vi "Begin.vi"() -> (1 "CameraDevRef":T5)   [LabVIEW 2011]
doc: "Called before other user functions, this VI is expected to open initial I/O refnums, load in file data, and do all program initialization. Notice that the <B>error out</B> terminal is simply used for data flow. Wiring it to other structures or subVIs ensures that this VI runs first."
uses:
  <vilib>/Rock Robotics/WPI/Camera/WPI_CameraDevRef.ctl
  <vilib>/Rock Robotics/WPI/Encoder/WPI_EncoderDevRef.ctl
  <vilib>/Rock Robotics/SystemInterfaces/Encoder/FPGA_EncoderIdx.ctl
  <vilib>/Rock Robotics/SystemInterfaces/Counter/FPGA_CounterCtrSystemIndex.ctl
  <vilib>/Rock Robotics/WPI/Encoder/WPI_EncoderType.ctl
  <vilib>/Rock Robotics/WPI/Joystick/WPI_JoystickDeviceEnum.ctl
  <vilib>/Rock Robotics/SystemInterfaces/DIO/FPGA_DIOPWMChannel.ctl
  <vilib>/Rock Robotics/SystemInterfaces/Typedef/FPGA_TypedefDigitalModule.ctl
  <vilib>/Rock Robotics/SystemInterfaces/DIO/FPGA_DIOChannel.ctl
  <vilib>/Rock Robotics/SystemInterfaces/AI/FPGA_AIChannel.ctl
  <vilib>/Rock Robotics/WPI/MotorControl/WPI_MotorControlOpen Victor.vi
  <vilib>/Rock Robotics/WPI/Counter/WPI_CounterDigitalInputToDigitalSource.vi
  Robot Global Data.vi
  <vilib>/Rock Robotics/WPI/MotorControl/WPI_MotorControlOpen Jaguar.vi
  <vilib>/Utility/file.llb/Read From Spreadsheet File (DBL).vi
  <vilib>/Rock Robotics/SystemInterfaces/DIO/FPGA_DIORelayChannel.ctl
  <vilib>/Rock Robotics/WPI/Relay/WPI_RelayDirection.ctl
  <vilib>/Rock Robotics/SystemInterfaces/AI/FPGA_AIGyroChannel.ctl
  <vilib>/Rock Robotics/SystemInterfaces/Typedef/FPGA_TypedefAnalogModule.ctl
panel:
  out "Path and file":string
  in  "Balls In Robot At Start":dbl=2.0
  out "EncoderDevRef 2":T1={"DevStatus"={"status"=FALSE, "code"=0, "source"=""}, "EncoderIndex"=enum."Invalid", "CounterIndex"=enum."Invalid", "DistancePerCount"=1.0, "Decoding Type"=enum."4x"}
  out "LDriveEncoder 2":errorcluster
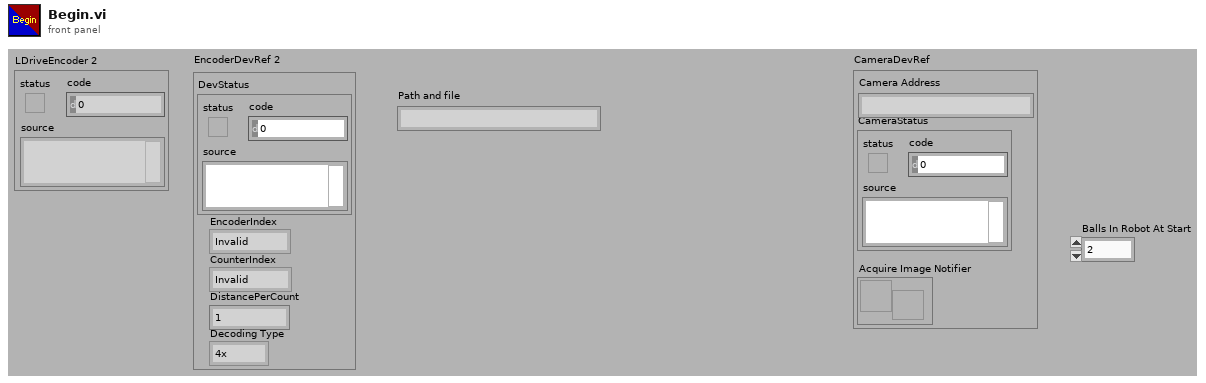
[diagram p1: front panel]
types:
  T1 = typedef "WPI_EncoderDevRef.ctl" = cluster{"DevStatus":errorcluster, "EncoderIndex":T2, "CounterIndex":T3, "DistancePerCount":dbl, "Decoding Type":T4}
  T2 = typedef "FPGA_EncoderIdx.ctl" = enum8{"Enc 0", "Enc 1", "Enc 2", "Enc 3", "Invalid"}
  T3 = typedef "FPGA_CounterCtrSystemIndex.ctl" = enum8{"Ctr 0", "Ctr 1", "Ctr 2", "Ctr 3", "Ctr 4", "Ctr 5", "Ctr 6", "Ctr 7", "Invalid"}
  T4 = typedef "WPI_EncoderType.ctl" = enum16{"1x", "2x", "4x"}
  T5 = typedef "WPI_CameraDevRef.ctl" = cluster{"Camera Address":string, "CameraStatus":errorcluster, "Acquire Image Notifier":refnum<notifier>}
  T6 = typedef "FPGA_DIOChannel.ctl" = enum8{"DIO 1", "DIO 2", "DIO 3", "DIO 4", "DIO 5", "DIO 6", "DIO 7", "DIO 8", "DIO 9", "DIO 10", "DIO 11", "DIO 12", "DIO 13", "DIO 14", "Invalid"}
  T7 = typedef "FPGA_DIOPWMChannel.ctl" = enum8{"PWM 1", "PWM 2", "PWM 3", "PWM 4", "PWM 5", "PWM 6", "PWM 7", "PWM 8", "PWM 9", "PWM 10", "Invalid"}
  T8 = typedef "FPGA_AIChannel.ctl" = enum8{"AI 1", "AI 2", "AI 3", "AI 4", "AI 5", "AI 6", "AI 7", "AI 8", "Invalid"}
  T9 = typedef "WPI_JoystickDeviceEnum.ctl" = enum16{"USB 1", "USB 2", "USB 3", "USB 4", "Kinect 1", "Kinect 2"}
  T10 = typedef "FPGA_TypedefDigitalModule.ctl" = enum16{"Digital Module 1", "Digital Module 2"}
  T11 = typedef "WPI_MotorControlDeviceRef.ctl" = cluster{"DeviceStatus":errorcluster, "Type":enum16{"PWM", "CAN"}, "PWM":cluster{"Digital Module":T10, "PWM Channel":T7, "DeadBand":T12}, "CAN":cluster{"Device Number":u8, "Control Mode":T13, "Semaphore":T14, "Max Vout":dbl}, "Invert":bool, "TransformRef":T15, "InvTransformRef":T15}
  T12 = typedef "WPI_PWMDeadband.ctl" = cluster{"Name":string, "maxPositivePwm":i32, "minPositivePwm":i32, "centerPwm":i32, "maxNegativePwm":i32, "minNegativePwm":i32, "angularRange":u16}
  T13 = typedef "WPI_CANJaguar_ControlMode.ctl" = enum8{"Percent VBus", "Current", "Speed", "Position", "Voltage"}
  T14 = typedef "Semaphore RefNum" = refnum<k1>
  T15 = typedef "WPI_PWMTransform_ConPane.ctl" = refnum<vi>
  T16 = typedef "WPI_CameraImageSize.ctl" = enum16{"640x480", "320x240", "160x120"}
  T17 = cluster{"fps":i32, "compression":i32, "Image Size":T16}
  T18 = typedef "WPI_CameraWhite Balance Values.ctl" = enum16{"Auto", "Fixed indoor", "Fixed outdoor 1", "Fixed outdoor 2", "Fixed fluorescent 1", "Fixed fluorescent 2", "Hold current"}
  T19 = typedef "WPI_CameraExposure Values.ctl" = enum16{"Auto", "Flicker-free 50 Hz", "Flicker-free 60 Hz", "Hold current"}
  T20 = typedef "WPI_ServoDeviceRef.ctl" = cluster{"DeviceStatus":errorcluster, "Digital Module":T10, "PWM Channel":T7, "DeadBand":T12}
  T21 = typedef "WPI_DigitalInputDevRef.ctl" = cluster{"DevStatus":errorcluster, "DIO Channel":T6, "Digital Module":T10}
  T22 = typedef "WPI_JoystickDevRef.ctl" = cluster{"Device":T9}
  T23 = typedef "FPGA_CounterEncoderSourceConvertionLVSourceType.ctl" = cluster{"DevStatus":errorcluster, "AnalogTriggerMode?":bool, "DigitalMode":cluster{"Digital Module":T10, "DIO Channel":T24}, "AnalogTriggerMode":cluster{"AnalogTriggerIndex":T25, "OutputType":T26}}
  T24 = typedef "FPGA_DIODigitalSourceChannel.ctl" = enum8{"DIO 1", "DIO 2", "DIO 3", "DIO 4", "DIO 5", "DIO 6", "DIO 7", "DIO 8", "DIO 9", "DIO 10", "DIO 11", "DIO 12", "DIO 13", "DIO 14", "Disabled"}
  T25 = typedef "FPGA_AnalogTriggerIndex.ctl" = enum8{"Trig 0", "Trig 1", "Trig 2", "Trig 3", "Trig 4", "Trig 5", "Trig 6", "Trig 7", "Invalid"}
  T26 = typedef "FPGA_AnalogTriggerOutType.ctl" = enum16{"InWindow", "TriggerState", "Rising", "Falling"}
  T27 = typedef "FPGA_DIORelayChannel.ctl" = enum8{"Relay 1", "Relay 2", "Relay 3", "Relay 4", "Relay 5", "Relay 6", "Relay 7", "Relay 8", "Invalid"}
  T28 = typedef "WPI_RelayDirection.ctl" = enum16{"Both directions", "Forward only", "Reverse only"}
  T29 = typedef "WPI_AnalogChannelDevRef.ctl" = cluster{"DevStatus":errorcluster, "Analog Module":T30, "Analog Channel":T8}
  T30 = typedef "FPGA_TypedefAnalogModule.ctl" = enum16{"Analog Module 1", "Analog Module 2"}
  T31 = typedef "WPI_RelayDevRef.ctl" = cluster{"DevStatus":errorcluster, "Relay Channel":T27, "Digital Module":T10, "Relay Direction":T28}
  T32 = typedef "FPGA_AIGyroChannel.ctl" = enum8{"AI 1", "AI 2", "Invalid"}
  T33 = typedef "WPI_GyroDevRef.ctl" = cluster{"DevStatus":errorcluster, "Analog Module":T30, "Analog Channel":T8, "Offset":dbl, "Gain (VoltsPerDegree/Second)":dbl}
  T34 = typedef "WPI_UltrasonicDeviceRef.ctl" = cluster{"DevStatus":errorcluster, "Ping Digital Module":T10, "Echo Digital Module":T10, "Ping Channel":T6, "Echo Channel":T6, "CntIndex":T3}
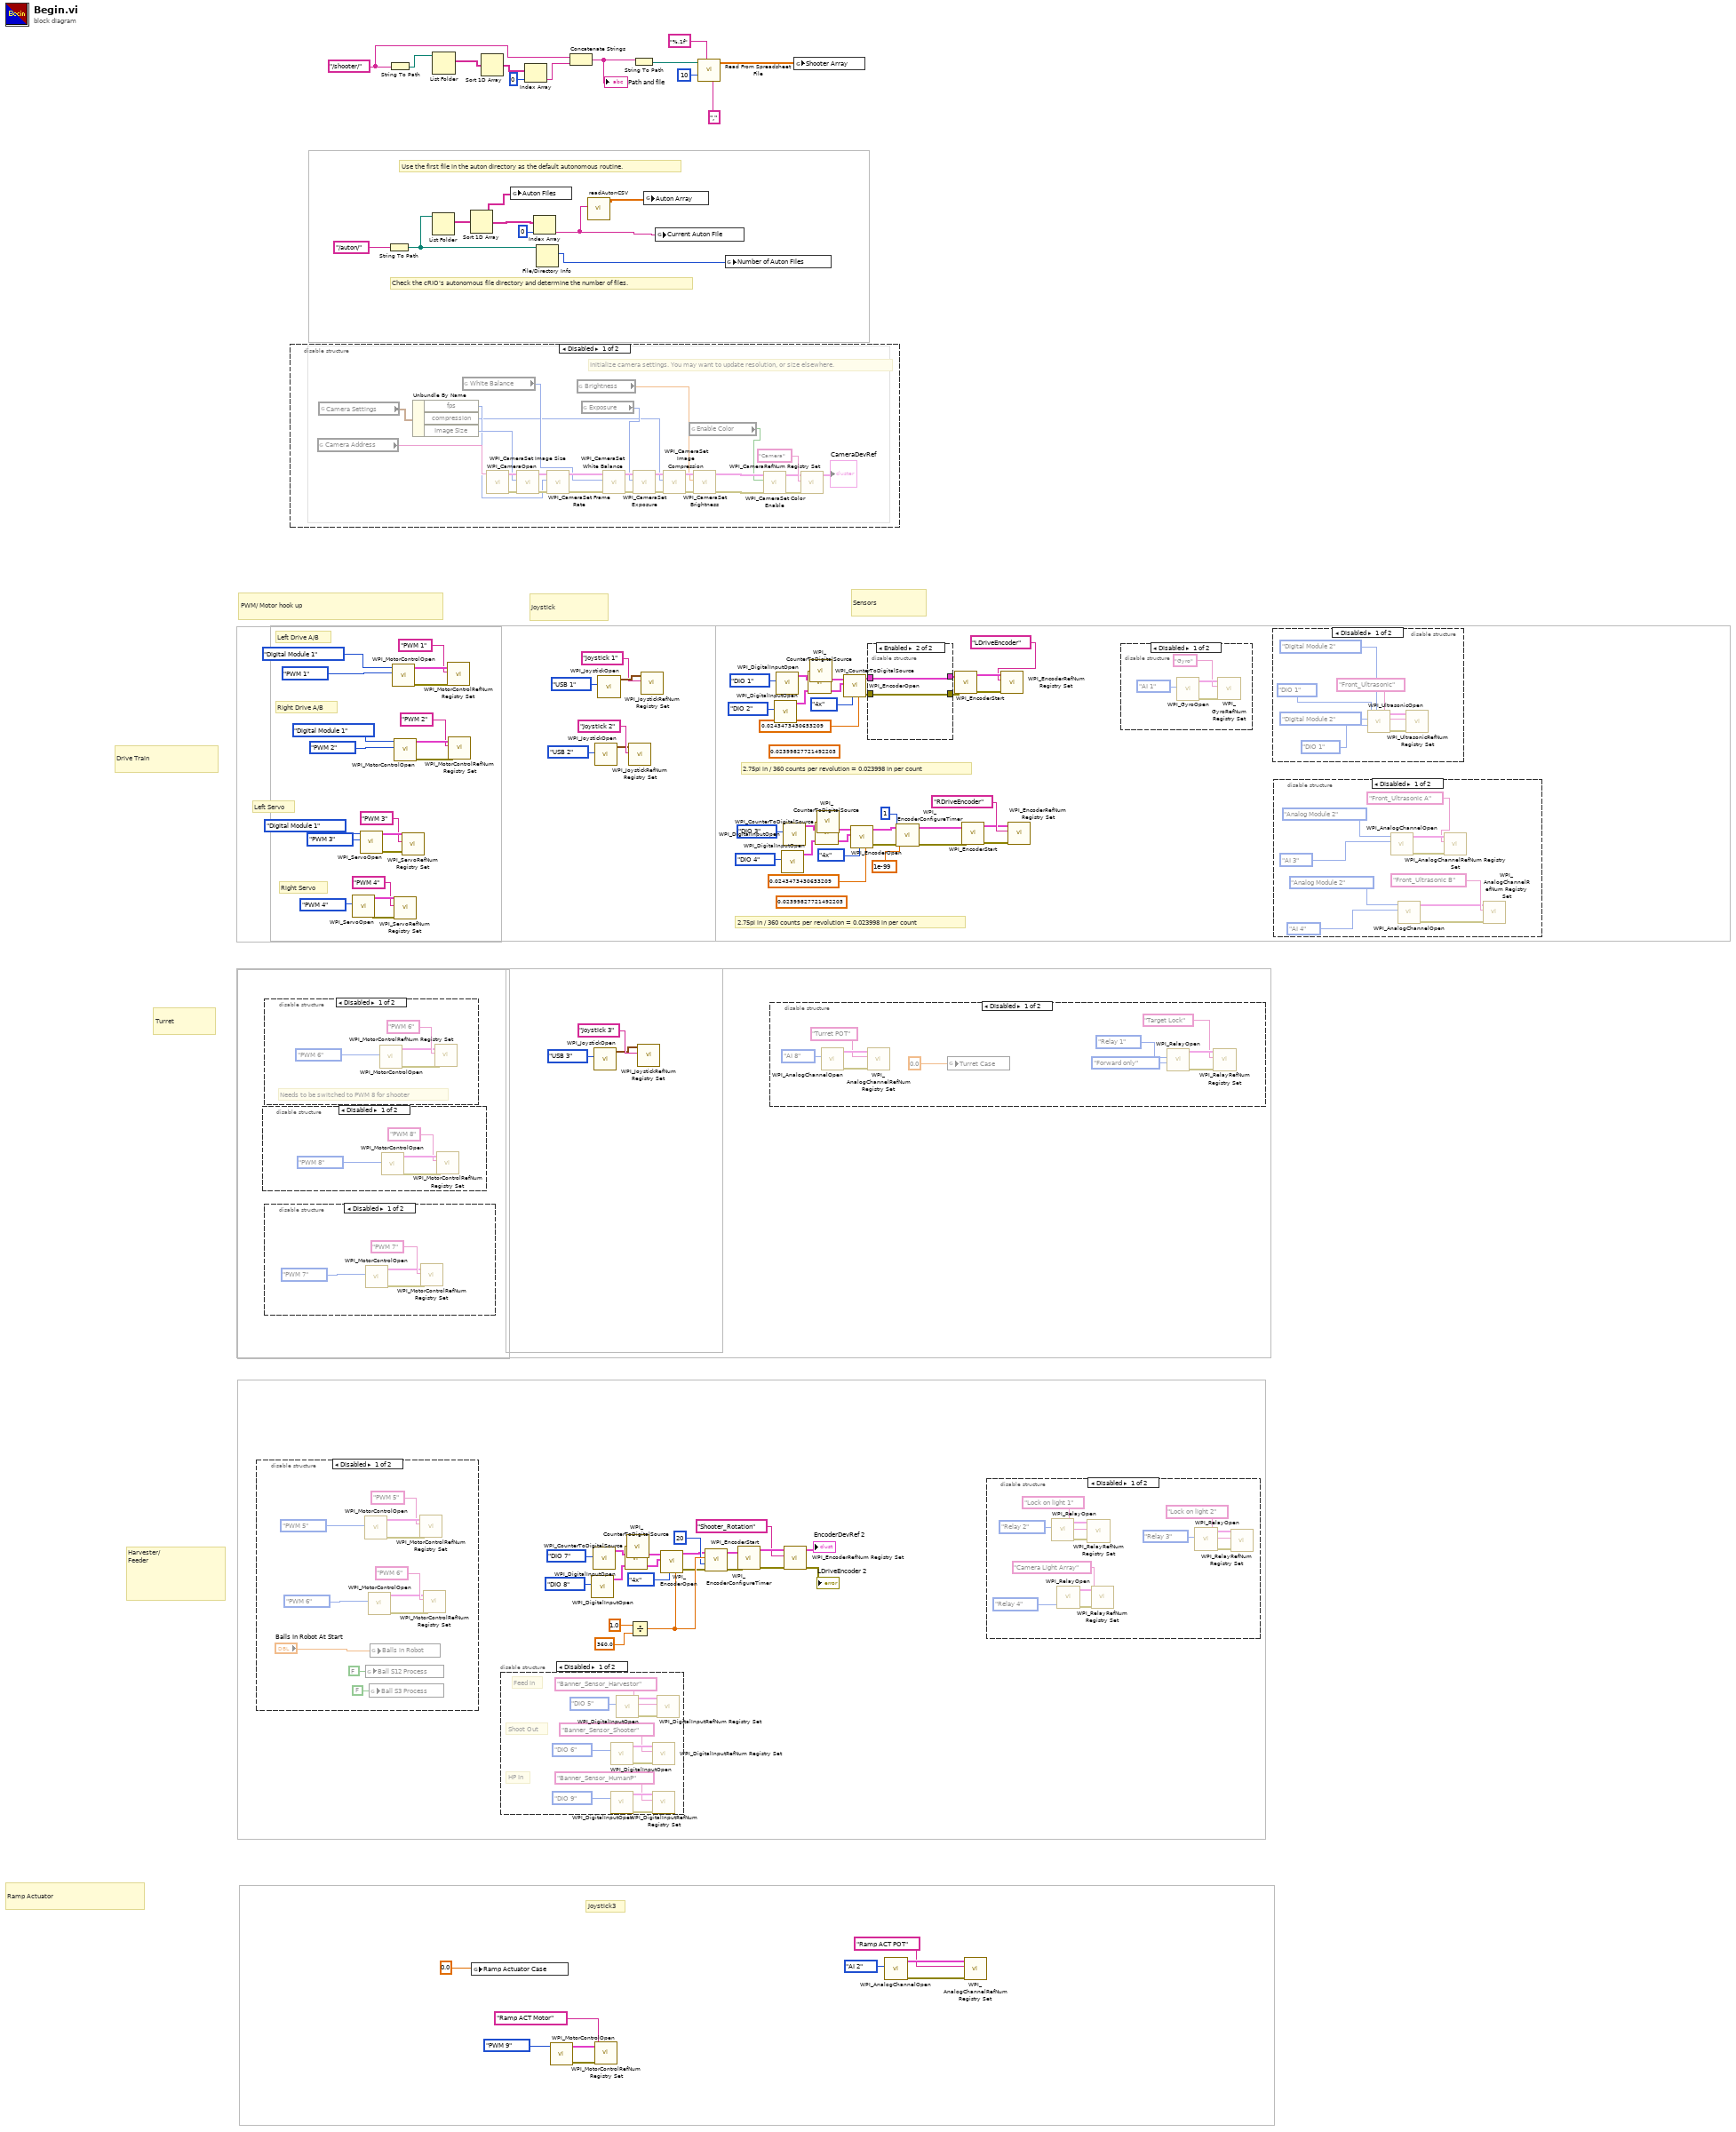
[diagram p0: block diagram]
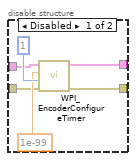
[diagram p2: hidden frame]
diagram:
  w26 = "/shooter/" ("string")
  (unwired) 0.02399827721492203 ("DistancePerCount")
  (unwired) 0.02399827721492203 ("DistancePerCount")
  # "2.75pi in / 360 counts per revolution = 0.023998 in per count"
  # "2.75pi in / 360 counts per revolution = 0.023998 in per count"
  # "Joystick3"
  # "Check the cRIO's autonomous file directory and determine the number of files."
  # "Use the first file in the auton directory as the default autonomous routine."
  # "Harvester/\nFeeder"
  # "Right Drive A/B"
  # "Left Drive A/B"
  # "Right Servo"
  # "Left Servo"
  # "Turret"
  # "Ramp Actuator"
  # "Drive Train"
  # "Sensors"
  # "Joystick"
  # "PWM/ Motor hook up"
  n1 = disable-structure shown="Disabled" {
    frame Disabled {
      n2 = call-poly <vilib>:"WPI_MotorControlOpen.vi"("PWM Channel"=FPGA_DIOPWMChannel."PWM 5") -> ("error out"=w117:errorcluster, "MotorControlDeviceRef"=w119:T11)  [unwired: 9 in]
      n3 = global write "Robot Global Data.vi" "Ball S12 Process"(FALSE ("Ball S12 Process")) -> ()
      n4 = call-poly <vilib>:"WPI_MotorControlOpen.vi"("PWM Channel"=FPGA_DIOPWMChannel."PWM 6") -> ("error out"=w116:errorcluster, "MotorControlDeviceRef"=w114:T11)  [unwired: 9 in]
      n5 = global write "Robot Global Data.vi" "Ball S3 Process"(FALSE ("Ball S3 Process")) -> ()
      n6 = global write "Robot Global Data.vi" "Balls in Robot"("Balls In Robot At Start") -> ()
      n7 = call <vilib>:"WPI_MotorControlRefNum Registry Set.vi"("error in (no error)"=w117, "refnum name"="PWM 5", "MotorControlDevRef"=w119) -> ()  [unwired: 7 in, 2 out]
      n8 = call <vilib>:"WPI_MotorControlRefNum Registry Set.vi"("error in (no error)"=w116, "refnum name"="PWM 6", "MotorControlDevRef"=w114) -> ()  [unwired: 7 in, 2 out]
    }
    frame Enabled {
    }
  }
  n9 = disable-structure shown="Disabled" {
    frame Disabled {
      n10 = call-poly <vilib>:"WPI_MotorControlOpen.vi"("PWM Channel"=FPGA_DIOPWMChannel."PWM 8") -> ("error out"=w121:errorcluster, "MotorControlDeviceRef"=w123:T11)  [unwired: 9 in]
      n11 = call <vilib>:"WPI_MotorControlRefNum Registry Set.vi"("error in (no error)"=w121, "refnum name"="PWM 8", "MotorControlDevRef"=w123) -> ()  [unwired: 7 in, 2 out]
    }
    frame Enabled {
    }
  }
  n12 = disable-structure shown="Disabled" {
    frame Disabled {
      # "Needs to be switched to PWM 8 for shooter"
      n13 = call-poly <vilib>:"WPI_MotorControlOpen.vi"("PWM Channel"=FPGA_DIOPWMChannel."PWM 6") -> ("error out"=w128:errorcluster, "MotorControlDeviceRef"=w126:T11)  [unwired: 9 in]
      n14 = call <vilib>:"WPI_MotorControlRefNum Registry Set.vi"("error in (no error)"=w128, "refnum name"="PWM 6", "MotorControlDevRef"=w126) -> ()  [unwired: 7 in, 2 out]
    }
    frame Enabled {
    }
  }
  n15 = disable-structure shown="Disabled" {
    frame Disabled {
      n16 = call-poly <vilib>:"WPI_MotorControlOpen.vi"("PWM Channel"=FPGA_DIOPWMChannel."PWM 7") -> ("error out"=w132:errorcluster, "MotorControlDeviceRef"=w130:T11)  [unwired: 9 in]
      n17 = call <vilib>:"WPI_MotorControlRefNum Registry Set.vi"("error in (no error)"=w132, "refnum name"="PWM 7", "MotorControlDevRef"=w130) -> ()  [unwired: 7 in, 2 out]
    }
    frame Enabled {
    }
  }
  n18 = disable-structure shown="Disabled" {
    frame Disabled {
      # "Initialize camera settings. You may want to update resolution, or size elsewhere."
      n19 = global read "Robot Global Data.vi" "Camera Address"() -> (w146:string)
      n20 = global read "Robot Global Data.vi" "Camera Settings"() -> (w145:T17)
      n21 = Unbundle By Name(w145) -> ("fps"=w143:i32, "compression"=w140:i32, "Image Size"=w144:T16)
      n22 = global read "Robot Global Data.vi" "White Balance"() -> (w142:T18)
      n23 = call <vilib>:"WPI_CameraOpen.vi"("Camera Address"=w146) -> ("error out"=w152:errorcluster, "CameraDevRef"=w153:T5)  [unwired: 1 in, 8 out]
      n24 = call <vilib>:"WPI_CameraSet Image Size.vi"("error in (no error)"=w152, "Image Size"=w144, "CameraDevRef"=w153) -> ("error out"=w151:errorcluster, "CameraDevRef Out"=w154:T5)  [unwired: 7 out]
      n25 = call <vilib>:"WPI_CameraSet Frame Rate.vi"("error in (no error)"=w151, "Frame Rate (fps)"=w143, "CameraDevRef"=w154) -> ("error out"=w150:errorcluster, "CameraDevRef Out"=w156:T5)  [unwired: 7 out]
      n26 = global read "Robot Global Data.vi" "Brightness"() -> (w139:dbl)
      n27 = global read "Robot Global Data.vi" "Exposure"() -> (w141:T19)
      n28 = call <vilib>:"WPI_CameraSet White Balance.vi"("error in (no error)"=w150, "White Balance"=w142, "CameraDevRef"=w156) -> ("error out"=w149:errorcluster, "CameraDevRef Out"=w155:T5)  [unwired: 7 out]
      n29 = call <vilib>:"WPI_CameraSet Exposure.vi"("error in (no error)"=w149, "Exposure"=w141, "CameraDevRef"=w155) -> ("error out"=w148:errorcluster, "CameraDevRef Out"=w158:T5)  [unwired: 7 out]
      n30 = call <vilib>:"WPI_CameraSet Image Compression.vi"("error in (no error)"=w148, "Compression"=w140, "CameraDevRef"=w158) -> ("error out"=w147:errorcluster, "CameraDevRef Out"=w157:T5)  [unwired: 7 out]
      n31 = global read "Robot Global Data.vi" "Enable Color"() -> (w134:bool)
      n32 = call <vilib>:"WPI_CameraSet Brightness.vi"("error in (no error)"=w147, "Brightness"=w139, "CameraDevRef"=w157) -> ("error out"=w137:errorcluster, "CameraDevRef Out"=w138:T5)  [unwired: 7 out]
      n33 = call <vilib>:"WPI_CameraSet Color Enable.vi"("error in (no error)"=w137, "Color Enabled"=w134, "CameraDevRef"=w138) -> ("error out"=w135:errorcluster, "CameraDevRef Out"=w136:T5)  [unwired: 7 in]
      n34 = call <vilib>:"WPI_CameraRefNum Registry Set.vi"("error in (no error)"=w135, "refnum name"="Camera", "CameraDevRef"=w136) -> ("CameraDevRef"=→"CameraDevRef":T5)  [unwired: 8 out]
    }
    frame Enabled {
    }
  }
  n35 = call <vilib>:"WPI_ServoOpen.vi"("PWM Channel"=FPGA_DIOPWMChannel."PWM 4") -> ("error out"=w85:errorcluster, "ServoDeviceRef"=w100:T20)  [unwired: 9 in]
  n36 = call <vilib>:"WPI_ServoOpen.vi"("PWM Channel"=FPGA_DIOPWMChannel."PWM 3", "Digital Module (Module 1)"=FPGA_TypedefDigitalModule."Digital Module 1") -> ("error out"=w86:errorcluster, "ServoDeviceRef"=w102:T20)  [unwired: 8 in]
  n37 = String To Path(string="/auton/") -> (path=w54:path)
  n38 = String To Path(string=w26) -> (path=w35:path)
  n39 = call-poly <vilib>:"WPI_MotorControlOpen.vi"("PWM Channel"=FPGA_DIOPWMChannel."PWM 1", "Digital Module (Module 1)"=FPGA_TypedefDigitalModule."Digital Module 1") -> ("error out"=w90:errorcluster, "MotorControlDeviceRef"=w93:T11)  [unwired: 8 in]
  n40 = call-poly <vilib>:"WPI_MotorControlOpen.vi"("PWM Channel"=FPGA_DIOPWMChannel."PWM 2", "Digital Module (Module 1)"=FPGA_TypedefDigitalModule."Digital Module 1") -> ("error out"=w91:errorcluster, "MotorControlDeviceRef"=w96:T11)  [unwired: 8 in]
  n41 = call <vilib>:"WPI_ServoRefNum Registry Set.vi"("error in (no error)"=w85, "refnum name"="PWM 4", "ServoDeviceRef"=w100) -> ()  [unwired: 7 in, 2 out]
  n42 = call <vilib>:"WPI_ServoRefNum Registry Set.vi"("error in (no error)"=w86, "refnum name"="PWM 3", "ServoDeviceRef"=w102) -> ()  [unwired: 7 in, 2 out]
  n43 = List Folder(path=w54) -> (filenames=w53:string[])  [unwired: 1 in, 5 out]
  n44 = List Folder(path=w35) -> (filenames=w34:string[])  [unwired: 1 in, 5 out]
  n45 = call <vilib>:"WPI_MotorControlRefNum Registry Set.vi"("error in (no error)"=w90, "refnum name"="PWM 1", "MotorControlDevRef"=w93) -> ()  [unwired: 7 in, 2 out]
  n46 = call <vilib>:"WPI_MotorControlRefNum Registry Set.vi"("error in (no error)"=w91, "refnum name"="PWM 2", "MotorControlDevRef"=w96) -> ()  [unwired: 7 in, 2 out]
  n47 = Sort 1D Array(array=w53) -> (sorted array=w48:string[])
  n48 = global write "Robot Global Data.vi" "Ramp Actuator Case"(0.0 ("Ramp Actuator Case")) -> ()
  n49 = Sort 1D Array(array=w34) -> (sorted array=w33:string[])
  n50 = disable-structure shown="Disabled" {
    frame Disabled {
      # "HP In"
      # "Shoot Out"
      # "Feed in"
      n51 = call <vilib>:"WPI_DigitalInputOpen.vi"("DIO Channel"=FPGA_DIOChannel."DIO 6") -> ("error out"=w166:errorcluster, "DigitalInputDevRef"=w165:T21)  [unwired: 9 in]
      n52 = call <vilib>:"WPI_DigitalInputOpen.vi"("DIO Channel"=FPGA_DIOChannel."DIO 9") -> ("error out"=w162:errorcluster, "DigitalInputDevRef"=w161:T21)  [unwired: 9 in]
      n53 = call <vilib>:"WPI_DigitalInputOpen.vi"("DIO Channel"=FPGA_DIOChannel."DIO 5") -> ("error out"=w169:errorcluster, "DigitalInputDevRef"=w168:T21)  [unwired: 9 in]
      n54 = call <vilib>:"WPI_DigitalInputRefNum Registry Set.vi"("error in (no error)"=w166, "refnum name"="Banner_Sensor_Shooter", "DigitalInputDevRef"=w165) -> ()  [unwired: 7 in, 2 out]
      n55 = call <vilib>:"WPI_DigitalInputRefNum Registry Set.vi"("error in (no error)"=w162, "refnum name"="Banner_Sensor_HumanP", "DigitalInputDevRef"=w161) -> ()  [unwired: 7 in, 2 out]
      n56 = call <vilib>:"WPI_DigitalInputRefNum Registry Set.vi"("error in (no error)"=w169, "refnum name"="Banner_Sensor_Harvestor", "DigitalInputDevRef"=w168) -> ()  [unwired: 7 in, 2 out]
    }
    frame Enabled {
    }
  }
  n57 = global write "Robot Global Data.vi" "Auton Files"(w48) -> ()
  n58 = Index Array(array=w33, index=0) -> (element=w25:string)
  n59 = Index Array(array=w48, index=0) -> (element=w50:string)
  n60 = File/Directory Info(path=w54) -> (size=w51:i64)  [unwired: 1 in, 6 out]
  n61 = call-poly <vilib>:"WPI_MotorControlOpen.vi"("PWM Channel"=FPGA_DIOPWMChannel."PWM 9") -> ("error out"=w38:errorcluster, "MotorControlDeviceRef"=w39:T11)  [unwired: 9 in]
  n62 = Concatenate Strings(w26, w25) -> (w28:string)
  "Path and file" <- w28
  n63 = call "readAutonCSV.vi"("AutonFile"=w50) -> ("AutonArray"=w49:dbl[][])  [unwired: 7 in]
  n64 = call <vilib>:"WPI_DigitalInputOpen.vi"("DIO Channel"=FPGA_DIOChannel."DIO 8") -> ("DigitalInputDevRef"=w8:T21)  [unwired: 9 in, 1 out]
  n65 = call <vilib>:"WPI_DigitalInputOpen.vi"("DIO Channel"=FPGA_DIOChannel."DIO 7") -> ("DigitalInputDevRef"=w5:T21)  [unwired: 9 in, 1 out]
  n66 = call <vilib>:"WPI_JoystickOpen.vi"("JoystickDevice"=WPI_JoystickDeviceEnum."USB 3") -> ("JoystickDevRef"=w46:T22)  [unwired: 10 in]
  n67 = call <vilib>:"WPI_JoystickOpen.vi"("JoystickDevice"=WPI_JoystickDeviceEnum."USB 2") -> ("JoystickDevRef"=w106:T22)  [unwired: 10 in]
  n68 = call <vilib>:"WPI_MotorControlRefNum Registry Set.vi"("error in (no error)"=w38, "refnum name"="Ramp ACT Motor", "MotorControlDevRef"=w39) -> ()  [unwired: 7 in, 2 out]
  n69 = call <vilib>:"WPI_JoystickOpen.vi"("JoystickDevice"=WPI_JoystickDeviceEnum."USB 1") -> ("JoystickDevRef"=w109:T22)  [unwired: 10 in]
  n70 = call-poly <vilib>:"WPI_CounterToDigitalSource.vi"("DigitalInputDevRef"=w8) -> ("Digital Source"=w9:T23)  [unwired: 6 in]
  n71 = call-poly <vilib>:"WPI_CounterToDigitalSource.vi"("DigitalInputDevRef"=w5) -> ("Digital Source"=w4:T23)  [unwired: 6 in]
  n72 = call <vilib>:"WPI_JoystickRefNum Registry Set.vi"("refnum name"="Joystick 2", "JoystickDevRef"=w106) -> ()  [unwired: 8 in, 2 out]
  n73 = Divide(x=1.0, y=360.0) -> (x/y=w23:dbl)
  n74 = String To Path(string=w28) -> (path=w27:path)
  n75 = call <vilib>:"WPI_JoystickRefNum Registry Set.vi"("refnum name"="Joystick 3", "JoystickDevRef"=w46) -> ()  [unwired: 8 in, 2 out]
  n76 = call <vilib>:"WPI_JoystickRefNum Registry Set.vi"("refnum name"="Joystick 1", "JoystickDevRef"=w109) -> ()  [unwired: 8 in, 2 out]
  n77 = global write "Robot Global Data.vi" "Auton Array"(w49) -> ()
  n78 = global write "Robot Global Data.vi" "Current Auton File"(w50) -> ()
  n79 = call <vilib>:"WPI_EncoderOpen.vi"("DistancePerCount"=w23, "Decoding Type"=WPI_EncoderType."4x", "BSource"=w9, "ASource"=w4) -> ("error out"=w12:errorcluster, "EncoderDevRef"=w13:T1)  [unwired: 6 in]
  n80 = call-poly <vilib>:"Read From Spreadsheet File.vi"("delimiter (\\t)"="," ("delimiter (\\t)"), "format (%.3f)"="%.1f", "number of rows (all:-1)"=10, "file path (dialog if empty)"=w27) -> ("all rows"=w24:dbl[][])  [unwired: 1 in, 6 out]
  n81 = call <vilib>:"WPI_EncoderConfigureTimer.vi"("error in (no error)"=w12, "Number Samples to Average"=u8 20, "Minimum Rate"=w23, "EncoderDevRef"=w13) -> ("error out"=w16:errorcluster, "EncoderDevRef"=w15:T1)  [unwired: 6 in]
  n82 = global write "Robot Global Data.vi" "Number of Auton Files"(w51) -> ()
  n83 = call <vilib>:"WPI_EncoderStart.vi"("error in (no error)"=w16, "EncoderDevRef"=w15) -> ("error out"=w18:errorcluster, "EncoderDevRef"=w17:T1)  [unwired: 8 in]
  n84 = disable-structure shown="Disabled" {
    frame Disabled {
      n85 = call <vilib>:"WPI_AnalogChannelOpen.vi"("Analog Channel"=FPGA_AIChannel."AI 8") -> ("error out"=w175:errorcluster, "AIDeviceRef"=w176:T29)  [unwired: 9 in]
      n86 = call <vilib>:"WPI_AnalogChannelRefNum Registry Set.vi"("error in (no error)"=w175, "refnum name"="Turret POT", "AIDeviceRef"=w176) -> ()  [unwired: 7 in, 2 out]
      n87 = global write "Robot Global Data.vi" "Turret Case"(0.0 ("Return To Home Case")) -> ()
      n88 = call <vilib>:"WPI_RelayOpen.vi"("Relay Direction"=WPI_RelayDirection."Forward only", "Relay Channel"=FPGA_DIORelayChannel."Relay 1") -> ("error out"=w180:errorcluster, "RelayDevRef"=w181:T31)  [unwired: 8 in]
      n89 = call <vilib>:"WPI_RelayRefNum Registry Set.vi"("error in (no error)"=w180, "refnum name"="Target Lock", "RelayDevRef"=w181) -> ()  [unwired: 7 in, 2 out]
    }
    frame Enabled {
    }
  }
  n90 = call <vilib>:"WPI_DigitalInputOpen.vi"("DIO Channel"=FPGA_DIOChannel."DIO 2") -> ("DigitalInputDevRef"=w76:T21)  [unwired: 9 in, 1 out]
  n91 = call <vilib>:"WPI_DigitalInputOpen.vi"("DIO Channel"=FPGA_DIOChannel."DIO 1") -> ("DigitalInputDevRef"=w73:T21)  [unwired: 9 in, 1 out]
  n92 = call <vilib>:"WPI_DigitalInputOpen.vi"("DIO Channel"=FPGA_DIOChannel."DIO 4") -> ("DigitalInputDevRef"=w67:T21)  [unwired: 9 in, 1 out]
  n93 = call <vilib>:"WPI_DigitalInputOpen.vi"("DIO Channel"=FPGA_DIOChannel."DIO 3") -> ("DigitalInputDevRef"=w70:T21)  [unwired: 9 in, 1 out]
  n94 = call <vilib>:"WPI_EncoderRefNum Registry Set.vi"("error in (no error)"=w18, "refnum name"="Shooter_Rotation", "EncoderDevRef"=w17) -> ("error out"=→"LDriveEncoder 2":errorcluster, "EncoderDevRef"=→"EncoderDevRef 2":T1)  [unwired: 7 in]
  n95 = global write "Robot Global Data.vi" "Shooter Array"(w24) -> ()
  n96 = call-poly <vilib>:"WPI_CounterToDigitalSource.vi"("DigitalInputDevRef"=w76) -> ("Digital Source"=w77:T23)  [unwired: 6 in]
  n97 = call-poly <vilib>:"WPI_CounterToDigitalSource.vi"("DigitalInputDevRef"=w73) -> ("Digital Source"=w72:T23)  [unwired: 6 in]
  n98 = call-poly <vilib>:"WPI_CounterToDigitalSource.vi"("DigitalInputDevRef"=w67) -> ("Digital Source"=w66:T23)  [unwired: 6 in]
  n99 = call-poly <vilib>:"WPI_CounterToDigitalSource.vi"("DigitalInputDevRef"=w70) -> ("Digital Source"=w71:T23)  [unwired: 6 in]
  n100 = call <vilib>:"WPI_EncoderOpen.vi"("DistancePerCount"=0.0243473430653209, "Decoding Type"=WPI_EncoderType."4x", "BSource"=w77, "ASource"=w72) -> ("error out"=w79:errorcluster, "EncoderDevRef"=w80:T1)  [unwired: 6 in]
  n101 = call <vilib>:"WPI_EncoderOpen.vi"("DistancePerCount"=0.0243473430653209, "Decoding Type"=WPI_EncoderType."4x", "BSource"=w66, "ASource"=w71) -> ("error out"=w63:errorcluster, "EncoderDevRef"=w62:T1)  [unwired: 6 in]
  n102 = disable-structure shown="Enabled" {
    disable-tunnel: [w187 w188] -> w82
    disable-tunnel: [w186 w189] -> w81
    disable-tunnel: w80 -> [w183 w189]
    disable-tunnel: w79 -> [w182 w188]
    frame Disabled {
      n103 = call <vilib>:"WPI_EncoderConfigureTimer.vi"("error in (no error)"=w182, "Number Samples to Average"=u8 1, "Minimum Rate"=1e-99, "EncoderDevRef"=w183) -> ("error out"=w187:errorcluster, "EncoderDevRef"=w186:T1)  [unwired: 6 in]
    }
    frame Enabled {
    }
  }
  n104 = call <vilib>:"WPI_AnalogChannelOpen.vi"("Analog Channel"=FPGA_AIChannel."AI 2") -> ("error out"=w43:errorcluster, "AIDeviceRef"=w44:T29)  [unwired: 9 in]
  n105 = call <vilib>:"WPI_EncoderConfigureTimer.vi"("error in (no error)"=w63, "Number Samples to Average"=u8 1, "Minimum Rate"=1e-99, "EncoderDevRef"=w62) -> ("error out"=w58:errorcluster, "EncoderDevRef"=w59:T1)  [unwired: 6 in]
  n106 = call <vilib>:"WPI_EncoderStart.vi"("error in (no error)"=w82, "EncoderDevRef"=w81) -> ("error out"=w84:errorcluster, "EncoderDevRef"=w83:T1)  [unwired: 8 in]
  n107 = call <vilib>:"WPI_EncoderStart.vi"("error in (no error)"=w58, "EncoderDevRef"=w59) -> ("error out"=w56:errorcluster, "EncoderDevRef"=w57:T1)  [unwired: 8 in]
  n108 = call <vilib>:"WPI_AnalogChannelRefNum Registry Set.vi"("error in (no error)"=w43, "refnum name"="Ramp ACT POT", "AIDeviceRef"=w44) -> ()  [unwired: 7 in, 2 out]
  n109 = disable-structure shown="Disabled" {
    frame Disabled {
      n110 = call <vilib>:"WPI_RelayOpen.vi"("Relay Channel"=FPGA_DIORelayChannel."Relay 2") -> ("error out"=w199:errorcluster, "RelayDevRef"=w198:T31)  [unwired: 9 in]
      n111 = call <vilib>:"WPI_RelayOpen.vi"("Relay Channel"=FPGA_DIORelayChannel."Relay 4") -> ("error out"=w201:errorcluster, "RelayDevRef"=w200:T31)  [unwired: 9 in]
      n112 = call <vilib>:"WPI_RelayRefNum Registry Set.vi"("error in (no error)"=w199, "refnum name"="Lock on light 1", "RelayDevRef"=w198) -> ()  [unwired: 7 in, 2 out]
      n113 = call <vilib>:"WPI_RelayRefNum Registry Set.vi"("error in (no error)"=w201, "refnum name"="Camera Light Array", "RelayDevRef"=w200) -> ()  [unwired: 7 in, 2 out]
      n114 = call <vilib>:"WPI_RelayOpen.vi"("Relay Channel"=FPGA_DIORelayChannel."Relay 3") -> ("error out"=w190:errorcluster, "RelayDevRef"=w191:T31)  [unwired: 9 in]
      n115 = call <vilib>:"WPI_RelayRefNum Registry Set.vi"("error in (no error)"=w190, "refnum name"="Lock on light 2", "RelayDevRef"=w191) -> ()  [unwired: 7 in, 2 out]
    }
    frame Enabled {
    }
  }
  n116 = call <vilib>:"WPI_EncoderRefNum Registry Set.vi"("error in (no error)"=w84, "refnum name"="LDriveEncoder", "EncoderDevRef"=w83) -> ()  [unwired: 7 in, 2 out]
  n117 = call <vilib>:"WPI_EncoderRefNum Registry Set.vi"("error in (no error)"=w56, "refnum name"="RDriveEncoder", "EncoderDevRef"=w57) -> ()  [unwired: 7 in, 2 out]
  n118 = disable-structure shown="Disabled" {
    frame Disabled {
      n119 = call <vilib>:"WPI_GyroOpen.vi"("Analog Channel"=FPGA_AIGyroChannel."AI 1") -> ("error out"=w205:errorcluster, "GyroDevRef"=w204:T33)  [unwired: 8 in, 1 out]
      n120 = call <vilib>:"WPI_GyroRefNum Registry Set.vi"("error in (no error)"=w205, "refnum name"="Gyro", "GyroDevRef"=w204) -> ()  [unwired: 7 in, 2 out]
    }
    frame Enabled {
    }
  }
  n121 = disable-structure shown="Disabled" {
    frame Disabled {
      n122 = call <vilib>:"WPI_UltrasonicOpen.vi"("Ping Digital Module (Module 1)"=FPGA_TypedefDigitalModule."Digital Module 2", "Echo DIO Channel"=FPGA_DIOChannel."DIO 1", "Echo Digital Module (Module 1)"=FPGA_TypedefDigitalModule."Digital Module 2", "Ping DIO Channel"=FPGA_DIOChannel."DIO 1") -> ("error out"=w212:errorcluster, "UltrasonicDevRef"=w211:T34)  [unwired: 6 in]
      n123 = call <vilib>:"WPI_UltrasonicRefNum Registry Set.vi"("error in (no error)"=w212, "refnum name"="Front_Ultrasonic", "UltrasonicDevRef"=w211) -> ()  [unwired: 7 in, 2 out]
    }
    frame Enabled {
    }
  }
  n124 = disable-structure shown="Disabled" {
    frame Disabled {
      n125 = call <vilib>:"WPI_AnalogChannelOpen.vi"("Analog Channel"=FPGA_AIChannel."AI 3", "Analog Module (Module 1)"=FPGA_TypedefAnalogModule."Analog Module 2") -> ("error out"=w218:errorcluster, "AIDeviceRef"=w217:T29)  [unwired: 8 in]
      n126 = call <vilib>:"WPI_AnalogChannelOpen.vi"("Analog Channel"=FPGA_AIChannel."AI 4", "Analog Module (Module 1)"=FPGA_TypedefAnalogModule."Analog Module 2") -> ("error out"=w213:errorcluster, "AIDeviceRef"=w214:T29)  [unwired: 8 in]
      n127 = call <vilib>:"WPI_AnalogChannelRefNum Registry Set.vi"("error in (no error)"=w218, "refnum name"="Front_Ultrasonic A", "AIDeviceRef"=w217) -> ()  [unwired: 7 in, 2 out]
      n128 = call <vilib>:"WPI_AnalogChannelRefNum Registry Set.vi"("error in (no error)"=w213, "refnum name"="Front_Ultrasonic B", "AIDeviceRef"=w214) -> ()  [unwired: 7 in, 2 out]
    }
    frame Enabled {
    }
  }
